vi "Write Record Data.vi"(8 "Error In (no error)":errorcluster, 10 "Record":variant, 11 "Expenses Tracker Category In":refnum<class "Expenses Tracker Category.lvclass">) -> (0 "Error Out":errorcluster, 3 "Expenses Tracker Category Out":refnum<class "Expenses Tracker Category.lvclass">)   [LabVIEW 2023, in "Expenses Tracker Category.lvclass"]
uses:
  Expenses Tracker Category.lvclass
  Expenses Tracker Record/Public/Ctrls/Category.ctl
  Expenses Tracker Category.lvclass/Expenses Tracker Category.ctl
  Expenses Tracker Record/Expenses Tracker Record.lvclass
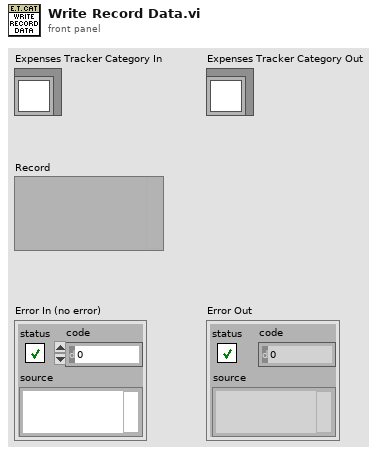
[diagram p1: front panel]
types:
  T1 = typedef "Expenses Tracker Record.lvclass/Category.ctl" = cluster{"ID":u32, "Name":string}
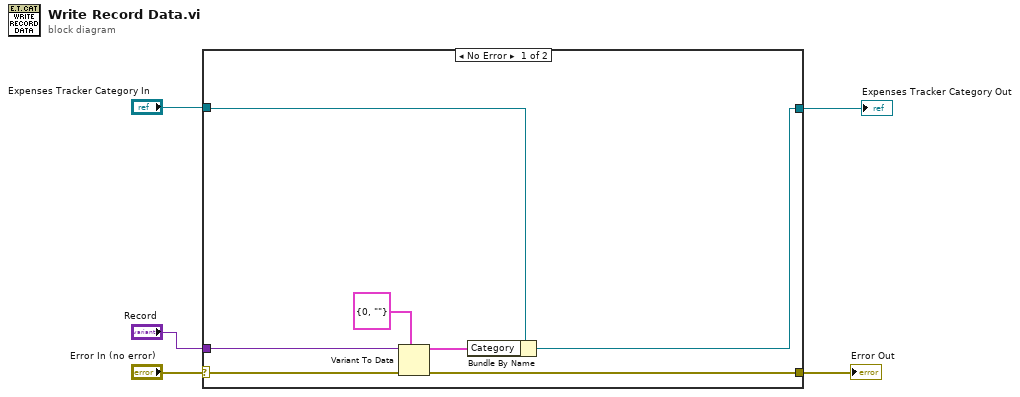
[diagram p0: block diagram]
diagram:
  n1 = case shown="No Error" "Error In (no error)" {
    selector: "Error In (no error)" -> [w10 w14]
    tunnel: [w8 w14] -> w4
    tunnel: [w6 w13] -> w3
    tunnel: "Expenses Tracker Category In" -> [w7 w13]
    tunnel: "Record" -> [w12 _]
    frame No Error {
      n2 = Variant To Data(error in=w10, type=T1 {"ID"=0, "Name"=""} ("Category"), Variant=w12) -> (data=w11:T1, error out=w8:errorcluster)
      n3 = Bundle By Name(cluster=w7, "Category"=w11) -> (w6:refnum<class "Expenses Tracker Category.lvclass">)
    }
    frame Error {
    }
  }
  "Error Out" <- w4
  "Expenses Tracker Category Out" <- w3
